vi "Meas.vi"(9 "input cluster":T1 {"Gain Coeff" format="%#_6e"; "Reserve 1" format="%02x"; "Mux TX/RX" format="%02x"; "ScanDelay" format="%02x"; "PacketCounter" format="%08x"; "SamplingInterval" format="%#_6e"; "Lose Packet" format="%08x"; "EncodersParam2" format="%016x"; "EncodersParam1" format="%016x"; "CRC 8" format="%02x"; "N chanel" format="%02x"; "N tick" format="%02x"; "Ncycle" format="%04x"; "FrameFormatVersion" format="%02x"; "MagicWord" format="%.0x"}, 10 "MeasControl":T2={"approx freq"=-1.0, "search (+/- % of Fsampl.)"=0.1, "start, duration"={"start samples/time"=0.0, "duration"=1.0, "EnableSubset"=FALSE}, "averaging type"=enum."Linear", "window"=enum."Rectangular (none)", "hysteresis"=0.0, "level"=0.0} {"level" format="%.2p"; "hysteresis" format="%.2p"; "start, duration"."duration" format="%0.2f"; "start, duration"."start samples/time" format="%0.2f"; "search (+/- % of Fsampl.)" format="%#_13g"}, 11 "signal_in":waveform(dbl)) -> (3 "Meas":T3 {"FFT amplitude mean" format="%.2p"; "DC" format="%0.2p"; "time trig 2" format="%0.2p"; "time trig" format="%0.2p"; "detected frequency 2" format="%.2p"; "way sensor 2" format="%.2p"; "way sensor 1" format="%.2p"; "detected frequency" format="%.2p"; "RMS" format="%0.2p"; "amplitude" format="%.2p"; "FFT amplitude" format="%.2p"})   [LabVIEW 2017]
uses:
  Control_EU/MeasControl.ctl
  Control_EU/MeasControl2.ctl
  Control_EU/UNDT_ClusterPackRevers (Type).ctl
  <vilib>/Waveform/WDTOps.llb/WDT Get Waveform Subset DBL.vi
  <vilib>/measure/matone.llb/Extract Single Tone Information 1 Chan.vi
  <vilib>/measure/mamon.llb/Trigger Detection for 1 Channel.vi
  <vilib>/measure/mascope.llb/Amplitude and Levels 1 chan.vi
  <vilib>/measure/madcrms.llb/Basic Averaged DC-RMS for 1 Chan.vi
  <vilib>/measure/NI_MAPro.lvlib
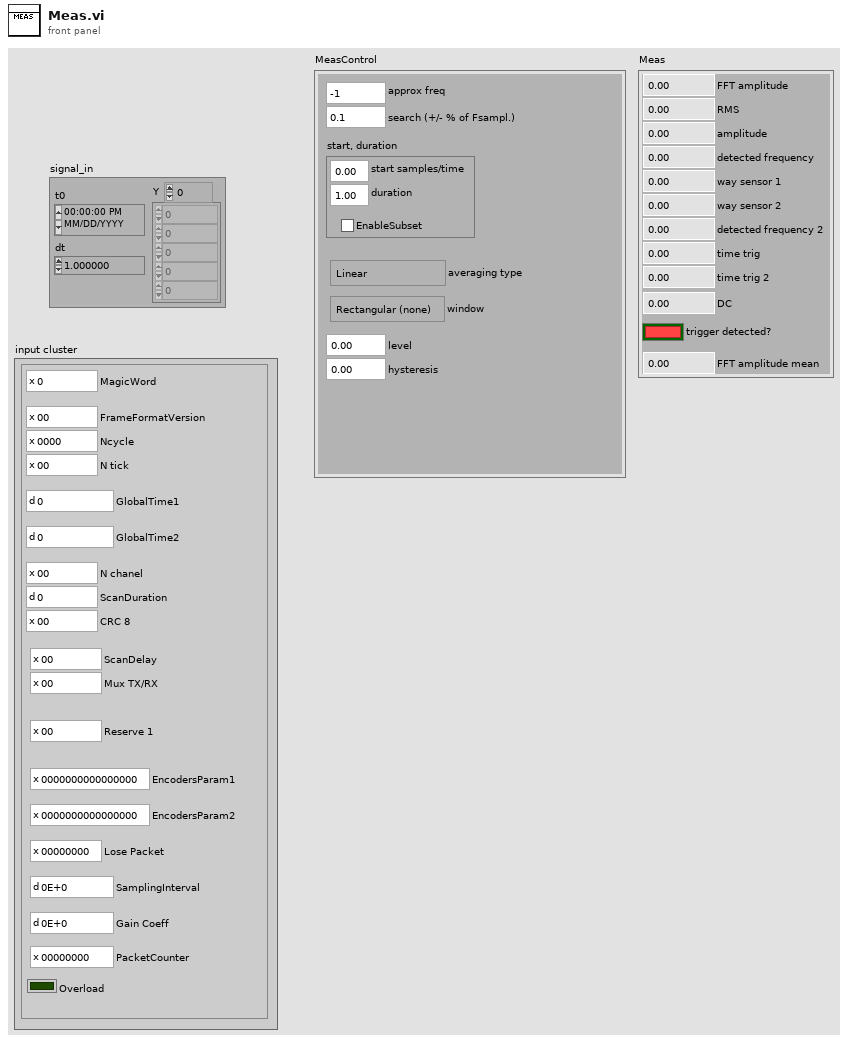
[diagram p1: front panel]
types:
  T1 = typedef "UNDT_ClusterPackRevers (Type).ctl" = cluster{"PacketCounter":u32, "Gain Coeff":sgl, "SamplingInterval":sgl, "Lose Packet":u32, "EncodersParam2":u64, "EncodersParam1":u64, "Reserve 1":u8, "Mux TX/RX":u8, "ScanDelay":u16, "CRC 8":u8, "ScanDuration":u16, "N chanel":u8, "GlobalTime2":u32, "GlobalTime1":u32, "N tick":u8, "Ncycle":u16, "FrameFormatVersion":u8, "MagicWord":u32, "Overload":bool}
  T2 = typedef "MeasControl2.ctl" = cluster{"approx freq":dbl, "search (+/- % of Fsampl.)":dbl, "start, duration":cluster{"start samples/time":dbl, "duration":dbl, "EnableSubset":bool}, "averaging type":enum16{"Linear", "Exponential"}, "window":enum16{"Rectangular (none)", "Hanning", "Low side lobe"}, "hysteresis":dbl, "level":dbl}
  T3 = typedef "MeasControl.ctl" = cluster{"FFT amplitude":dbl, "amplitude":dbl, "RMS":dbl, "detected frequency":dbl, "way sensor 1":ext, "way sensor 2":ext, "detected frequency 2":dbl, "time trig":dbl, "time trig 2":dbl, "DC":dbl, "trigger detected?":bool, "FFT amplitude mean":dbl}
  T4 = cluster{"approx freq. (optional)":dbl, "search (+/- % of Fsampl.)":dbl}
  T5 = cluster{"start samples/time":dbl, "duration":dbl, "EnableSubset":bool}
  T6 = enum16{"Rectangular (none)", "Hanning", "Low side lobe"}
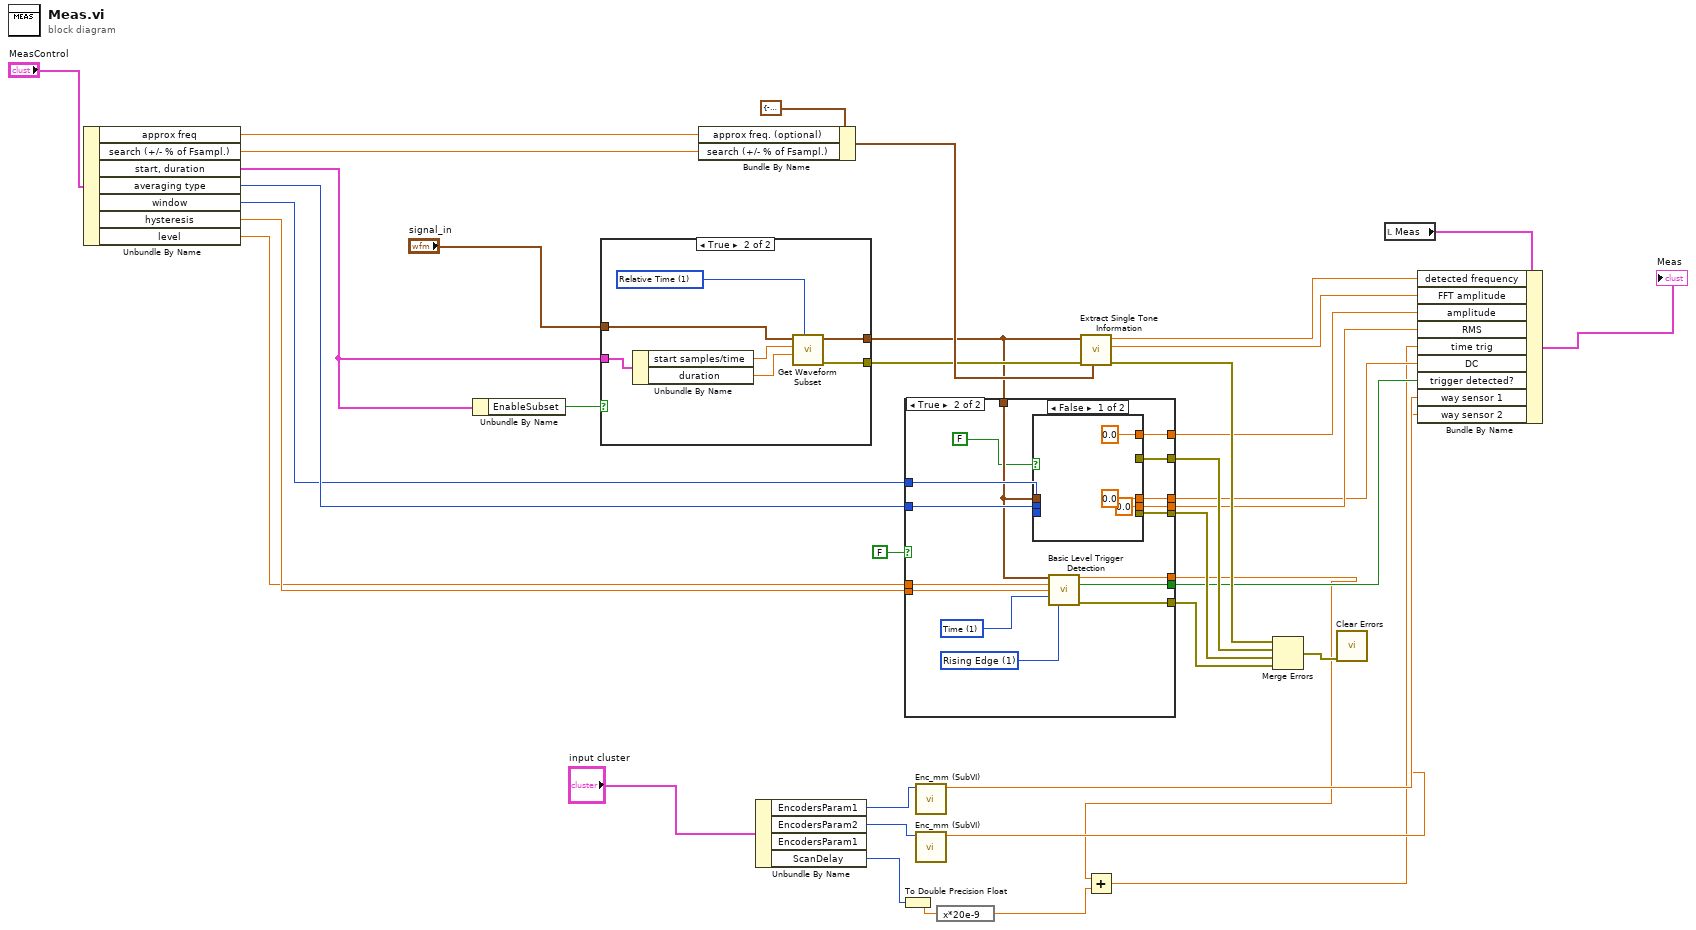
[diagram p0: block diagram]
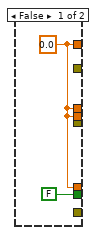
[diagram p2: hidden frame]
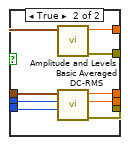
[diagram p3: hidden frame]
diagram:
  n1 = Unbundle By Name("MeasControl") -> ("approx freq"=w22:dbl, "search (+/- % of Fsampl.)"=w21:dbl, "start, duration"=w20:T5, "averaging type"=w19:enum16{"Linear", "Exponential"}, "window"=w18:T6, "hysteresis"=w17:dbl, "level"=w16:dbl)
  n2 = Unbundle By Name(w20) -> ("EnableSubset"=w30:bool)
  n3 = case shown="True" w30 {
    tunnel: "signal_in" -> [w39 w46]
    tunnel: [w39 w42] -> w13
    tunnel: w20 -> [_ w41]
    tunnel: [_ w40] -> w14
    frame False {
    }
    frame True {
      w45 = u16 1 items=["Samples", "Relative Time"] ("start/duration format")
      n4 = Unbundle By Name(w41) -> ("start samples/time"=w44:dbl, "duration"=w43:dbl)
      n5 = call-poly <vilib>:"Get Waveform Subset.vi"("start/duration format"=w45, "duration"=w43, "start samples/time"=w44, "waveform in"=w46) -> ("error out"=w40:errorcluster, "waveform out"=w42:waveform(dbl))  [unwired: 2 in, 2 out]
    }
  }
  n6 = Bundle By Name(cluster=T4 {"approx freq. (optional)"=-1.0, "search (+/- % of Fsampl.)"=1.0} ("advanced search"), "approx freq. (optional)"=w22, "search (+/- % of Fsampl.)"=w21) -> (w15:T4)
  n7 = Unbundle By Name("input cluster") -> ("EncodersParam1"=w9:u64, "EncodersParam2"=w10:u64, "ScanDelay"=w3:u16)  [unwired: 1 out]
  n8 = To Double Precision Float(number=w3) -> (double precision float=w5:dbl)
  n9 = case shown="True" FALSE {
    tunnel: [_ w64] -> w32
    tunnel: [_ w63] -> w31
    tunnel: [w48 w62] -> w28
    tunnel: [w48 w61] -> w27
    tunnel: [_ w58] -> w26
    tunnel: [w48 w57] -> w2
    tunnel: [w48 w56] -> w25
    tunnel: [FALSE ("trigger detected?") w55] -> w24
    tunnel: w19 -> [_ w54]
    tunnel: w18 -> [_ w53]
    tunnel: w17 -> [_ w52]
    tunnel: w16 -> [_ w51]
    tunnel: w13 -> [_ w50]
    frame False {
      w48 = 0.0 ("amplitude")
    }
    frame True {
      w59 = u16 1 items=["Falling Edge", "Rising Edge"] ("trigger slope")
      w60 = u16 1 items=["Index", "Time"] ("location mode")
      n10 = case shown="False" FALSE {
        tunnel: [_ w75] -> w64
        tunnel: [_ w74] -> w63
        tunnel: [0.0 ("amplitude") w73] -> w62
        tunnel: [0.0 ("RMS value") w72] -> w61
        tunnel: [0.0 ("DC value") w71] -> w56
        tunnel: w54 -> [_ w70]
        tunnel: w53 -> [_ w69]
        tunnel: w50 -> [_ w68]
        frame False {
        }
        frame True {
          n11 = call-poly <vilib>:"Amplitude and Levels.vi"("signal in"=w68) -> ("error out"=w75:errorcluster, "amplitude"=w73:dbl)  [unwired: 7 in, 2 out]
          n12 = call-poly <vilib>:"Basic Averaged DC-RMS.vi"("window"=w69, "averaging type"=w70, "signal in"=w68) -> ("error out"=w74:errorcluster, "RMS value"=w72:dbl, "DC value"=w71:dbl)  [unwired: 5 in, 1 out]
        }
      }
      n13 = call-poly <vilib>:"Basic Level Trigger Detection.vi"("signal in"=w50, "level"=w51, "hysteresis"=w52, "location mode"=w60, "trigger slope"=w59) -> ("trigger location"=w57:dbl, "trigger detected?"=w55:bool, "error out"=w58:errorcluster)  [unwired: 8 in]
    }
  }
  n14 = call "Enc_mm (SubVI).vi"("EncodersParam1"=w9) -> ("Numeric"=w8:ext)  [unwired: 10 in]
  n15 = call "Enc_mm (SubVI).vi"("EncodersParam1"=w10) -> ("Numeric"=w7:ext)  [unwired: 10 in]
  n16 = expression code="x*20e-9"(w5) -> (w4:dbl)
  n17 = call-poly <vilib>:"Extract Single Tone Information.vi"("advanced search"=w15, "error in (no error)"=w14, "time signal in"=w13) -> ("error out"=w37:errorcluster, "detected amplitude"=w29:dbl, "detected frequency"=w33:dbl)  [unwired: 3 in, 3 out]
  n18 = Add(x=w2, y=w4) -> (x+y=w1:dbl)
  n19 = Merge Errors(w37, w32, w31, w26) -> (w35:errorcluster)
  n20 = call <vilib>:"Clear Errors.vi"("error in (no error)"=w35) -> ()  [unwired: 5 in, 2 out]
  n21 = local read "Meas"() -> (w36:T3)
  n22 = Bundle By Name(cluster=w36, "detected frequency"=w33, "FFT amplitude"=w29, "amplitude"=w28, "RMS"=w27, "time trig"=w1, "DC"=w25, "trigger detected?"=w24, "way sensor 1"=w8, "way sensor 2"=w7) -> (→"Meas":T3)
